vi "문자형.vi"() -> ()   [LabVIEW 2020]
panel:
  out "연결된 문자열":string
  in  "멪음말":string
  in  "머리말":string
  out "합계":string
  out "결과":dbl
  in  "D":dbl
  in  "C":i32
  in  "B":dbl
  in  "A":dbl
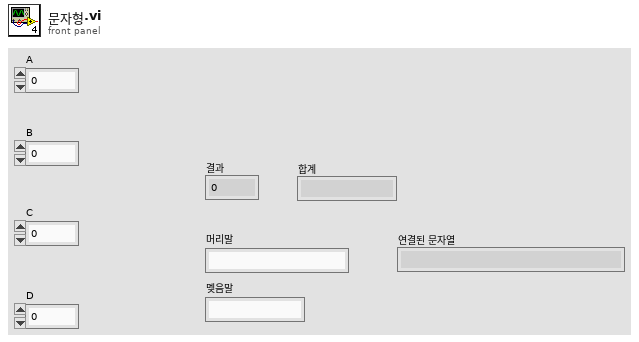
[diagram p1: front panel]
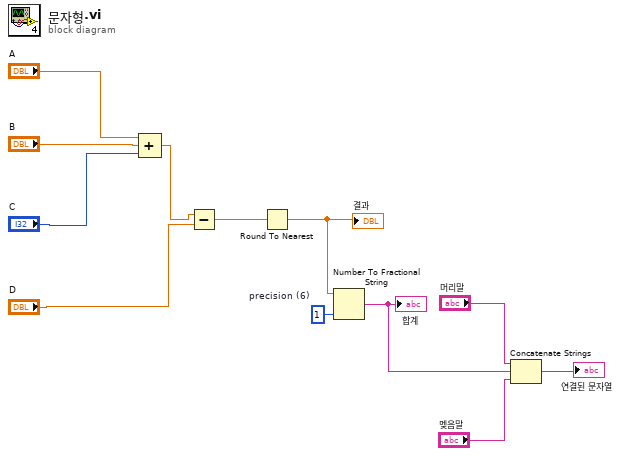
[diagram p0: block diagram]
diagram:
  w5 = i16 1  # precision (6)
  n1 = Compound Arithmetic op=ADD("A", "B", "C") -> (w9:dbl)
  n2 = Subtract(x=w9, y="D") -> (x-y=w7:dbl)
  n3 = Round To Nearest(number=w7) -> (nearest integer value=w6:dbl)
  "결과" <- w6
  n4 = Number To Fractional String(number=w6, precision (6)=w5) -> (F-format string=w4:string)  [unwired: 2 in]
  "합계" <- w4
  n5 = Concatenate Strings("머리말", w4, "멪음말") -> (→"연결된 문자열":string)
